vi "检测有效.vi"(3 "一维数组":dbl[](array[numeric]), 4 "按键数组":bool[][](array[boolean]), 5 "空的位置":dbl=8.0) -> (0 "空的坐标":cluster{"x":i32, "y":i32}, 1 "按键位置":cluster{"x":i32, "y":i32}, 2 "有效":bool)   [LabVIEW 2009]
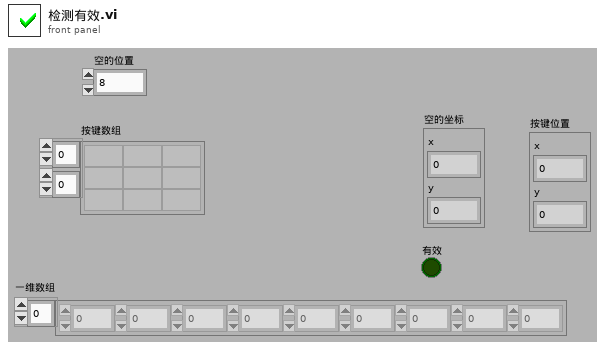
[diagram p1: front panel]
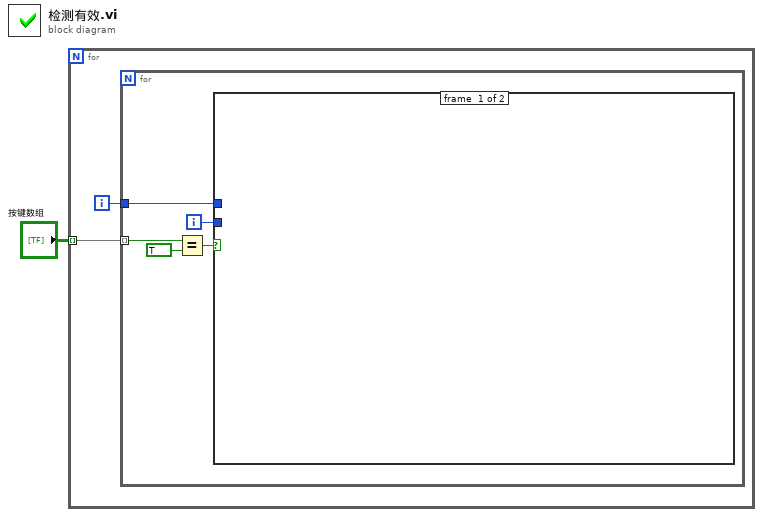
[diagram p0: block diagram]
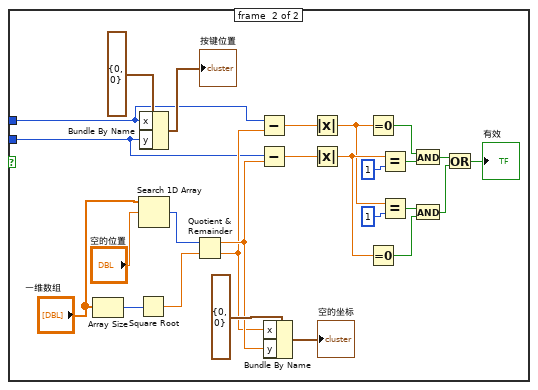
[diagram p2: hidden frame]
diagram:
  n1 = for {
    tunnel: "按键数组" -> [w3] mode=indexing
    i -> [w2]
    n2 = for {
      tunnel: w3 -> [w8] mode=indexing
      tunnel: w2 -> [w4]
      i -> [w5]
      n3 = Equal?(x=w8, y=TRUE) -> (x = y?=w6:bool)
      n4 = case shown="真" w6 {
        tunnel: w5 -> [_ w9]
        tunnel: w4 -> [_ w10]
        frame #0 {
        }
        frame #1 {
          n5 = Array Size(array="一维数组") -> (size(s)=w18:i32)
          n6 = Square Root(x=w18) -> (sqrt(x)=w20:dbl)
          n7 = Search 1D Array(1D array="一维数组", element="空的位置") -> (index of element=w12:i32)  [unwired: 1 in]
          n8 = Bundle By Name(cluster=cluster{"x":i32, "y":i32} {"x"=0, "y"=0}, "x"=w10, "y"=w9) -> (→"按键位置":cluster{"x":i32, "y":i32})
          n9 = Quotient & Remainder(x=w12, y=w20) -> (x-y*floor(x/y)=w15:dbl, floor(x/y)=w14:dbl)
          n10 = Subtract(x=w10, y=w14) -> (x-y=w21:dbl)
          n11 = Subtract(x=w9, y=w15) -> (x-y=w22:dbl)
          n12 = Bundle By Name(cluster=cluster{"x":i32, "y":i32} {"x"=0, "y"=0}, "x"=w14, "y"=w15) -> (→"空的坐标":cluster{"x":i32, "y":i32})
          n13 = Absolute Value(x=w21) -> (abs(x)=w25:dbl)
          n14 = Absolute Value(x=w22) -> (abs(x)=w26:dbl)
          n15 = Equal To 0?(x=w25) -> (x = 0?=w27:bool)
          n16 = Equal To 0?(x=w26) -> (x = 0?=w30:bool)
          n17 = Equal?(x=w26, y=1) -> (x = y?=w28:bool)
          n18 = Equal?(x=w25, y=1) -> (x = y?=w29:bool)
          n19 = And(x=w27, y=w28) -> (x .and. y?=w31:bool)
          n20 = And(x=w29, y=w30) -> (x .and. y?=w32:bool)
          n21 = Or(x=w31, y=w32) -> (x .or. y?=→"有效":bool)
        }
      }
    }
  }
